vi "car_CarWash_main.vi"(7 "Command (Check Car Wash Cycle)":T4=enum."Check Car Wash Cycle", 8 "error in (no error)":errorcluster, 10 "Car Wash Simulation Switches":T2, 11 "Purchase Selection":T3) -> (0 "error out":errorcluster, 2 "Completed Car Wash":bool, 3 "Car Wash Indicators":T1)   [LabVIEW 2009]
doc: "This VI is the main VI for the Car Wash module. This VI contains the logic and state information for move from one Car Wash state to another.\n\nSee Block Diagram for detailed information."
uses:
  car_CarWash_Command_enum.ctl
  car_CarWash_PurchaseSelection_enum.ctl
  controls/car_CarWashSimulationSwitches_cluster.ctl
  controls/car_CarWashIndicators_cluster.ctl
  car_CarWash_CycleTimes_cluster.ctl
  timer/car_Timer_Command_enum.ctl
  car_CarWash_Cycles_enum.ctl
panel:
  # "Inputs"
  # "Outputs"
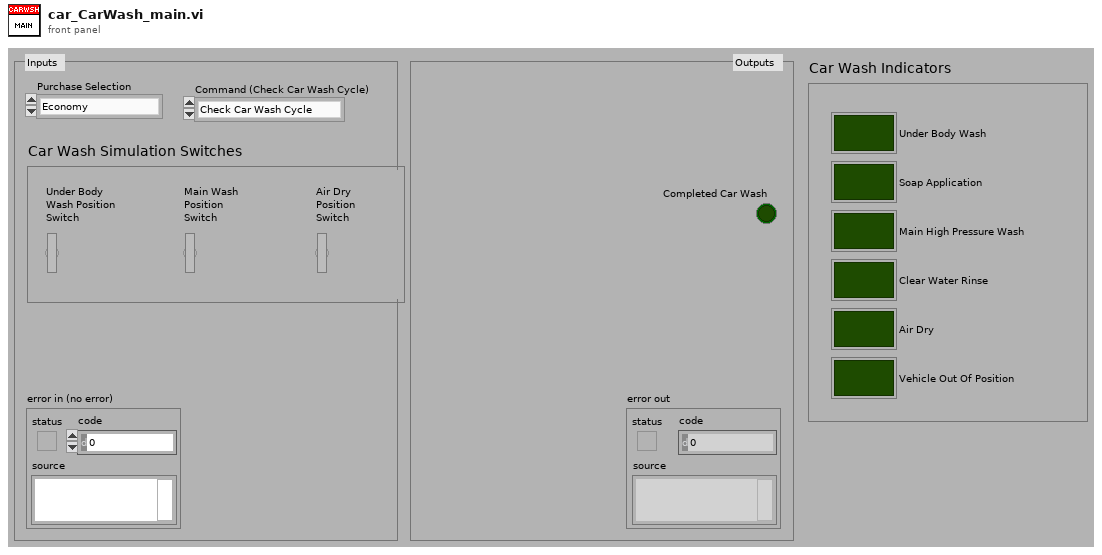
[diagram p1: front panel]
types:
  T1 = typedef "car_CarWashIndicators_cluster.ctl" = cluster{"Under Body Wash":bool, "Soap Application":bool, "Main High Pressure Wash":bool, "Clear Water Rinse":bool, "Air Dry":bool, "Vehicle Out Of Position":bool}
  T2 = typedef "car_CarWashSimulationSwitches_cluster.ctl" = cluster{"Under Body Wash Position Switch":bool, "Main Wash Position Switch":bool, "Air Dry Position Switch":bool}
  T3 = typedef "car_CarWash_PurchaseSelection_enum.ctl" = enum16{"Economy", "Deluxe"}
  T4 = typedef "car_CarWash_Command_enum.ctl" = enum16{"Initialise", "Start Car Wash", "Check Car Wash Cycle", "Next Cycle", "Shutdown"}
  T5 = typedef "car_CarWash_CycleTimes_cluster.ctl" = cluster{"Underbody Wash":dbl, "Soap Application":dbl, "Main High-Pressure Wash":dbl, "Clear Water Rinse":dbl, "Air Dry":dbl}
  T6 = typedef "car_Timer_Command_enum.ctl" = enum16{"Start Timer", "Check Timer"}
  T7 = typedef "car_CarWash_Cycles_enum.ctl" = enum16{"Underbody Wash", "Soap Application", "Main High-Pressure Wash", "Clear Water Rinse", "Air Dry Cycle"}
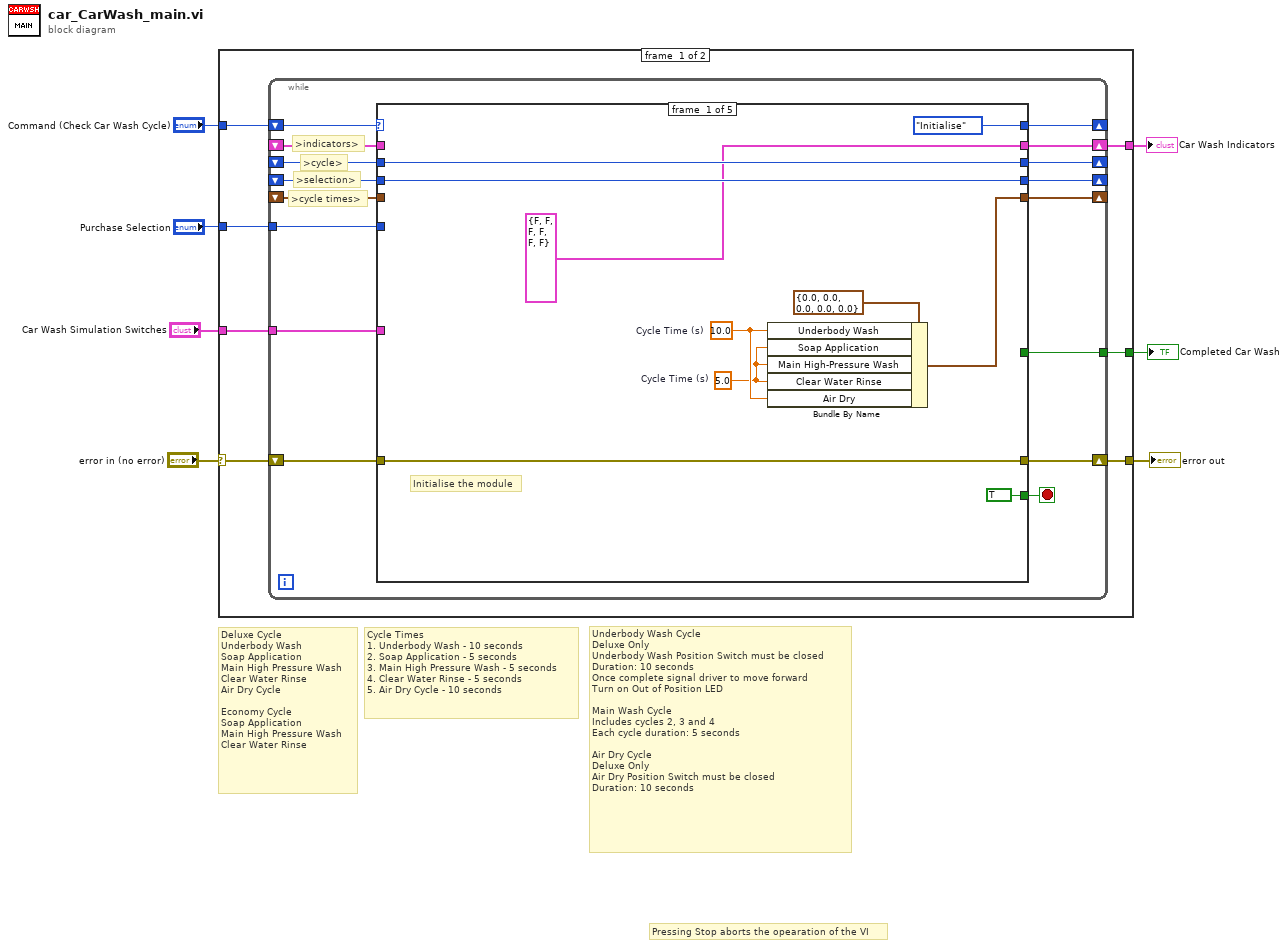
[diagram p0: block diagram]
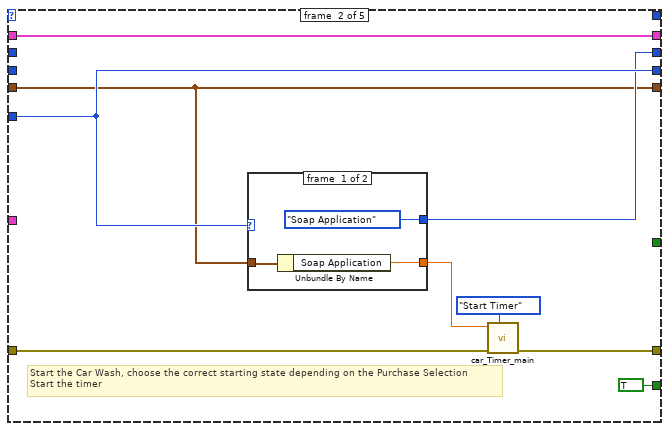
[diagram p2: hidden frame]
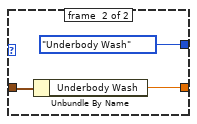
[diagram p3: hidden frame]
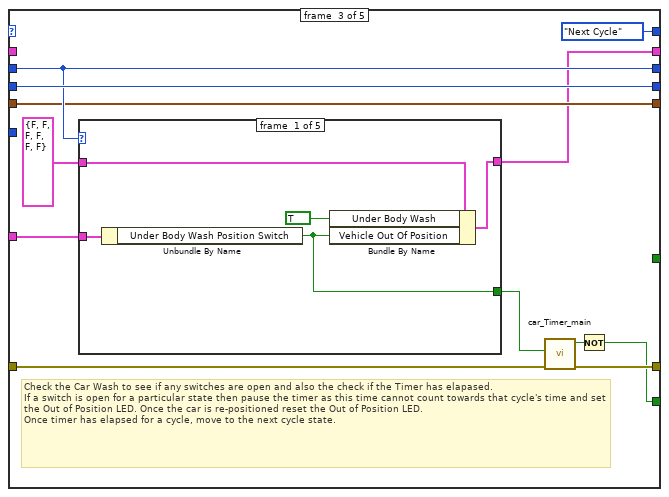
[diagram p4: hidden frame]
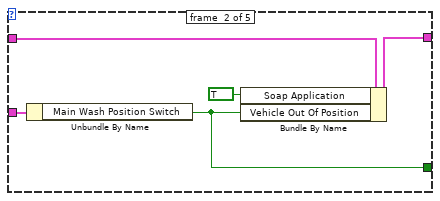
[diagram p5: hidden frame]
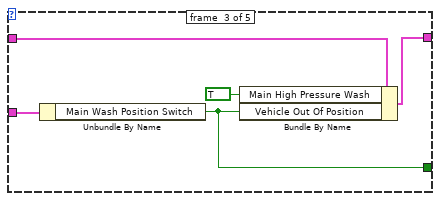
[diagram p6: hidden frame]
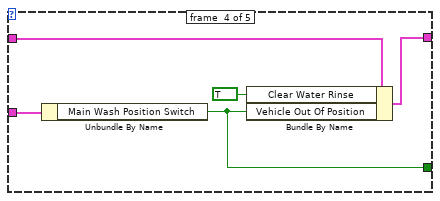
[diagram p7: hidden frame]
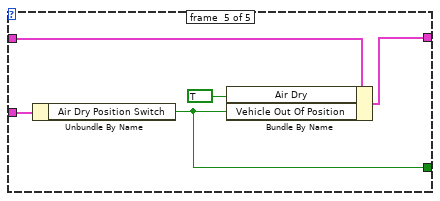
[diagram p8: hidden frame]
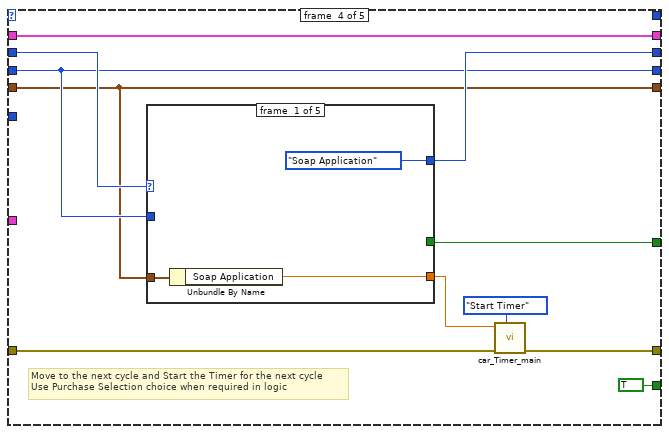
[diagram p9: hidden frame]
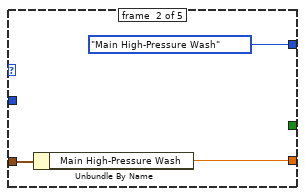
[diagram p10: hidden frame]
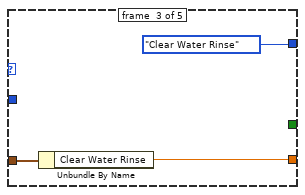
[diagram p11: hidden frame]
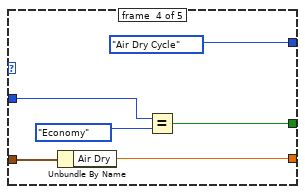
[diagram p12: hidden frame]
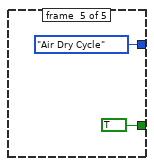
[diagram p13: hidden frame]
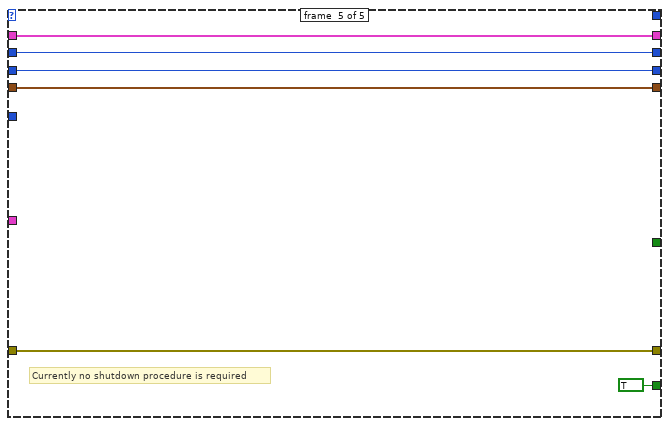
[diagram p14: hidden frame]
diagram:
  # "Pressing Stop aborts the opearation of the VI"
  # "Underbody Wash Cycle\nDeluxe Only\nUnderbody Wash Position Switch must be closed\nDuration: 10 seconds\nOnce complete signal driver to move forward\nTurn on Out of Position LED\n\nMain Wash Cycle\nIncludes cycles 2, 3 and 4\nEach cycle duration: 5 seconds\n\nAir Dry Cycle\nDeluxe Only\nAir Dry Position Switch must be closed\nDuration: 10 seconds"
  # "Cycle Times\n1. Underbody Wash - 10 seconds\n2. Soap Application - 5 seconds\n3. Main High Pressure Wash - 5 seconds\n4. Clear Water Rinse - 5 seconds\n5. Air Dry Cycle - 10 seconds"
  # "Deluxe Cycle\nUnderbody Wash\nSoap Application\nMain High Pressure Wash\nClear Water Rinse\nAir Dry Cycle\n\nEconomy Cycle\nSoap Application\nMain High Pressure Wash\nClear Water Rinse"
  n1 = case shown="No Error" "error in (no error)" {
    selector: "error in (no error)" -> [w14 w127]
    tunnel: [w13 w127] -> w5
    tunnel: "Command (Check Car Wash Cycle)" -> [w10 _]
    tunnel: "Purchase Selection" -> [w12 _]
    tunnel: "Car Wash Simulation Switches" -> [w11 _]
    tunnel: [w9 _] -> w2
    tunnel: [w8 _] -> w1
    frame #0 {
      n2 = while {
        shift-right: [w30] -> w13
        shift-left: w14 -> [w29]
        shift-right: [w28] -> _
        shift-left: _ -> [w27]
        shift-right: [w26] -> _
        shift-left: _ -> [w25]
        tunnel: w12 -> [w24]
        shift-right: [w23] -> _
        shift-left: _ -> [w22]
        tunnel: w11 -> [w21]
        shift-right: [w18] -> _
        shift-left: w10 -> [w19]
        shift-right: [w17] -> w8
        shift-left: _ -> [w16]
        tunnel: [w15] -> w9
        stop <- w20 stop-if-true
        # ">indicators>"
        # ">cycle times>"
        # ">selection>"
        # ">cycle>"
        n3 = case shown="\"Next Cycle\"" w19 {
          tunnel: [w40 w43 w59 w96 w126] -> w30
          tunnel: w29 -> [w40 w44 w60 w97 w126]
          tunnel: [w34 w48 w66 w101 w125] -> w28
          tunnel: w27 -> [w34 _ w66 w102 w125]
          tunnel: [w35 w49 w67 w98 w124] -> w26
          tunnel: w25 -> [w35 _ w67 w98 w124]
          tunnel: w24 -> [_ w49 _ _ _]
          tunnel: [w38 w42 w65 w94 w123] -> w23
          tunnel: w22 -> [_ w42 w65 w94 w123]
          tunnel: w21 -> [_ _ w64 _ _]
          tunnel: [TRUE TRUE w57 TRUE TRUE] -> w20
          tunnel: [car_CarWash_Command_enum."Initialise" ("Command (Check Car Wash Cycle)") _ car_CarWash_Command_enum."Next Cycle" ("Command (Check Car Wash Cycle)") _ _] -> w18
          tunnel: [T1 {"Under Body Wash"=FALSE, "Soap Application"=FALSE, "Main High Pressure Wash"=FALSE, "Clear Water Rinse"=FALSE, "Air Dry"=FALSE, "Vehicle Out Of Position"=FALSE} ("Car Wash Indicators") w46 w61 w103 w121] -> w17
          tunnel: w16 -> [_ w46 _ w103 w121]
          tunnel: [_ _ _ w100 _] -> w15
          frame #0 {
            w36 = 5.0  # Cycle Time (s)
            w37 = 10.0  # Cycle Time (s)
            # "Initialise the module"
            n4 = Bundle By Name(cluster=T5 {"Underbody Wash"=0.0, "Soap Application"=0.0, "Main High-Pressure Wash"=0.0, "Clear Water Rinse"=0.0, "Air Dry"=0.0} ("Cycle Times"), "Underbody Wash"=w37, "Soap Application"=w36, "Main High-Pressure Wash"=w36, "Clear Water Rinse"=w36, "Air Dry"=w37) -> (w38:T5)
          }
          frame #1 {
            # "Start the Car Wash, choose the correct starting state depending on the Purchase Selection\nStart the timer"
            n5 = case shown="\"Economy\"" w49 {
              tunnel: [car_CarWash_Cycles_enum."Soap Application" ("Car Wash Cycles") car_CarWash_Cycles_enum."Underbody Wash" ("Car Wash Cycles")] -> w48
              tunnel: w42 -> [w51 w54]
              tunnel: [w50 w53] -> w41
              frame #0 {
                n6 = Unbundle By Name(w51) -> ("Soap Application"=w50:dbl)
              }
              frame #1 {
                n7 = Unbundle By Name(w54) -> ("Underbody Wash"=w53:dbl)
              }
            }
            n8 = call "car_Timer_main.vi"("Command (Check Timer)"=car_Timer_Command_enum."Start Timer", "error in (no error)"=w44, "Target Time (s)"=w41) -> ("error out"=w43:errorcluster)  [unwired: 7 in, 1 out]
          }
          frame #2 {
            # "Check the Car Wash to see if any switches are open and also the check if the Timer has elapased.\nIf a switch is open for a particular state then pause the timer as this time cannot count towards that cycle's time and set the Out of Position LED. Once the car is re-positioned reset the Out of Position LED.\nOnce timer has elapsed for a cycle, move to the next cycle state."
            n9 = case shown="\"Underbody Wash\"" w66 {
              tunnel: w64 -> [w72 w77 w82 w87 w92]
              tunnel: [w69 w75 w79 w85 w90] -> w56
              tunnel: T1 {"Under Body Wash"=FALSE, "Soap Application"=FALSE, "Main High Pressure Wash"=FALSE, "Clear Water Rinse"=FALSE, "Air Dry"=FALSE, "Vehicle Out Of Position"=FALSE} ("Car Wash Indicators") -> [w71 w76 w81 w86 w91]
              tunnel: [w70 w74 w80 w83 w88] -> w61
              frame #0 {
                n10 = Unbundle By Name(w72) -> ("Under Body Wash Position Switch"=w69:bool)
                n11 = Bundle By Name(cluster=w71, "Under Body Wash"=TRUE, "Vehicle Out Of Position"=w69) -> (w70:T1)
              }
              frame #1 {
                n12 = Unbundle By Name(w77) -> ("Main Wash Position Switch"=w75:bool)
                n13 = Bundle By Name(cluster=w76, "Soap Application"=TRUE, "Vehicle Out Of Position"=w75) -> (w74:T1)
              }
              frame #2 {
                n14 = Unbundle By Name(w82) -> ("Main Wash Position Switch"=w79:bool)
                n15 = Bundle By Name(cluster=w81, "Main High Pressure Wash"=TRUE, "Vehicle Out Of Position"=w79) -> (w80:T1)
              }
              frame #3 {
                n16 = Unbundle By Name(w87) -> ("Main Wash Position Switch"=w85:bool)
                n17 = Bundle By Name(cluster=w86, "Clear Water Rinse"=TRUE, "Vehicle Out Of Position"=w85) -> (w83:T1)
              }
              frame #4 {
                n18 = Unbundle By Name(w92) -> ("Air Dry Position Switch"=w90:bool)
                n19 = Bundle By Name(cluster=w91, "Air Dry"=TRUE, "Vehicle Out Of Position"=w90) -> (w88:T1)
              }
            }
            n20 = call "car_Timer_main.vi"("error in (no error)"=w60, "Pause"=w56) -> ("error out"=w59:errorcluster, "Elapsed"=w58:bool)  [unwired: 8 in]
            n21 = Not(x=w58) -> (.not. x?=w57:bool)
          }
          frame #3 {
            # "Move to the next cycle and Start the Timer for the next cycle\nUse Purchase Selection choice when required in logic"
            n22 = case shown="\"Air Dry Cycle\"" w102 {
              tunnel: [car_CarWash_Cycles_enum."Soap Application" ("Car Wash Cycles") car_CarWash_Cycles_enum."Main High-Pressure Wash" ("Car Wash Cycles") car_CarWash_Cycles_enum."Clear Water Rinse" ("Car Wash Cycles") car_CarWash_Cycles_enum."Air Dry Cycle" ("Car Wash Cycles") car_CarWash_Cycles_enum."Air Dry Cycle" ("Car Wash Cycles")] -> w101
              tunnel: [_ _ _ w115 TRUE] -> w100
              tunnel: w98 -> [_ _ _ w117 _]
              tunnel: w94 -> [w105 w108 w111 w114 _]
              tunnel: [w104 w107 w110 w113 _] -> w93
              frame #0 {
                n23 = Unbundle By Name(w105) -> ("Soap Application"=w104:dbl)
              }
              frame #1 {
                n24 = Unbundle By Name(w108) -> ("Main High-Pressure Wash"=w107:dbl)
              }
              frame #2 {
                n25 = Unbundle By Name(w111) -> ("Clear Water Rinse"=w110:dbl)
              }
              frame #3 {
                n26 = Unbundle By Name(w114) -> ("Air Dry"=w113:dbl)
                n27 = Equal?(x=w117, y=car_CarWash_PurchaseSelection_enum."Economy") -> (x = y?=w115:bool)
              }
              frame #4 {
              }
            }
            n28 = call "car_Timer_main.vi"("Command (Check Timer)"=car_Timer_Command_enum."Start Timer", "error in (no error)"=w97, "Target Time (s)"=w93) -> ("error out"=w96:errorcluster)  [unwired: 7 in, 1 out]
          }
          frame #4 {
            # "Currently no shutdown procedure is required"
          }
        }
      }
    }
    frame #1 {
    }
  }
  "error out" <- w5
  "Car Wash Indicators" <- w1
  "Completed Car Wash" <- w2
